vi "Pre Launch Init.vi"(11 "DLS Laser Actor in":refnum<class "FLS Laser Actor.lvclass">) -> (0 "error out":errorcluster, 3 "DLS Laser Actor out":refnum<class "FLS Laser Actor.lvclass">)   [LabVIEW 2018, in "FLS Laser Actor.lvlib" / "FLS Laser Actor.lvclass"]
doc: "Sends a high priority message to it's self to notify the monitor that it's spawned. If it's in the runtime environment, this message is never sent, meaning the monitor will never spawn\n\nCopyright: MGI\nAuthored by: Derek Trepanier"
uses:
  FLS Laser Actor.lvclass
  FLS Laser Actor.lvclass/FLS Laser Actor.ctl
  Actor Monitor/Actor/Monitored Actor.lvclass
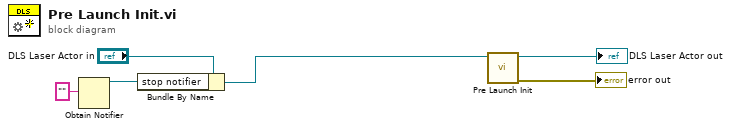
[diagram p0: block diagram]
diagram:
  n1 = Obtain Notifier(notification data type="") -> (notifier out=w2:refnum<notifier>)  [unwired: 3 in, 2 out]
  n2 = Bundle By Name(cluster="DLS Laser Actor in", "stop notifier"=w2) -> (w1:refnum<class "FLS Laser Actor.lvclass">)
  n3 = call-parent "Pre Launch Init.vi"("Monitored Actor in"=w1) -> ("error out"=→"error out":errorcluster, "Monitored Actor out"=→"DLS Laser Actor out":refnum<class "FLS Laser Actor.lvclass">)  [unwired: 9 in]
